vi "Write Server RPC Methods.vi"(8 "error in (no error)":errorcluster, 10 "Server RPC Methods":T1, 11 "ServiceName Template in":refnum<class "ServiceName Template.lvclass">) -> (0 "error out":errorcluster, 3 "ServiceName Template out":refnum<class "ServiceName Template.lvclass">)   [LabVIEW 2024, in "ServiceName Template.lvclass"]
uses:
  ServiceName Template.lvclass
  typeDefs/Server gRPC UEs.ctl
  gRPC lv Support/grpc-lvsupport/gRPCId Cluster.ctl
  gRPC lv Support/grpc-lvsupport/grpcId.ctl
  ServiceName Template.lvclass/ServiceName Template.ctl
  gRPC lv Support/grpc-lvsupport/grpc-lvsupport.lvlib
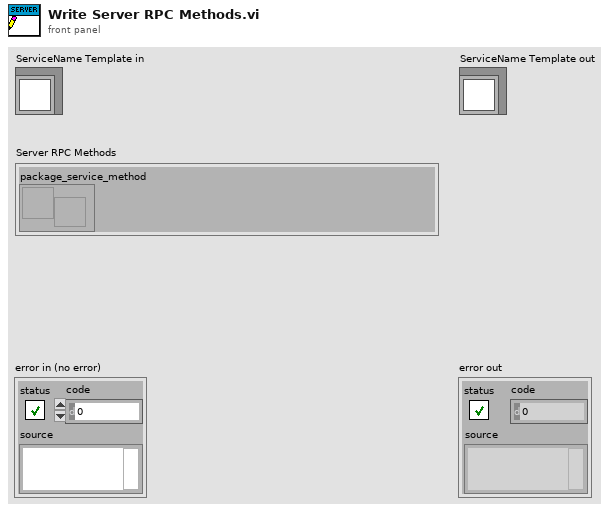
[diagram p1: front panel]
types:
  T1 = typedef "ServiceName Template.lvclass/Server gRPC UEs.ctl" = cluster{"package_service_method":refnum<user-event>}
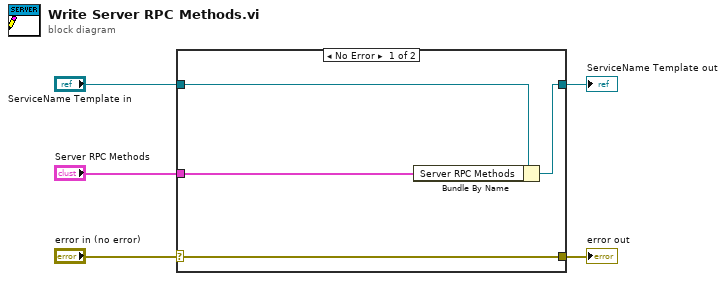
[diagram p0: block diagram]
diagram:
  n1 = case shown="No Error" "error in (no error)" {
    selector: "error in (no error)" -> [w9 w10]
    tunnel: [w9 w10] -> w4
    tunnel: [w7 w11] -> w2
    tunnel: "ServiceName Template in" -> [w8 w11]
    tunnel: "Server RPC Methods" -> [w6 _]
    frame No Error {
      n2 = Bundle By Name(cluster=w8, "Server RPC Methods"=w6) -> (w7:refnum<class "ServiceName Template.lvclass">)
    }
    frame Error {
    }
  }
  "error out" <- w4
  "ServiceName Template out" <- w2
